vi "Channel Path.vi"(10 "Variant":variant) -> (1 "Channel Library Path":path, 3 "Channel Folder Path":path)   [LabVIEW 2022 SP3, in "FlexBlocks Support.lvlib"]
uses:
  FlexBlocks Support.lvlib
  <resource>/ChannelSupport/_ChannelScriptingSupport/_ChannelScriptingSupport.lvlib
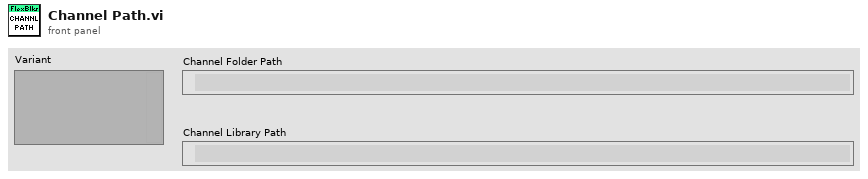
[diagram p1: front panel]
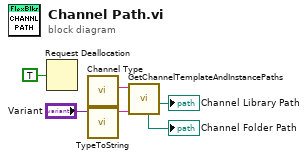
[diagram p0: block diagram]
diagram:
  n1 = Request Deallocation(TRUE ("flag")) -> ()
  n2 = call "Channel Type.vi"() -> ("Channel Template"=w1:string)  [unwired: 11 in]
  n3 = call <resource>:"TypeToString.vi"("type"="Variant") -> ("string"=w6:string)  [unwired: 10 in]
  n4 = call <resource>:"GetChannelTemplateAndInstancePaths.vi"("element typestring"=w6, "channel kind"=w1) -> ("cached channel instance library path"=→"Channel Library Path":path, "cached channel instance library elements path"=→"Channel Folder Path":path)  [unwired: 4 in, 4 out]
